vi "CH_LM Calibration Password.vi"(0 "Meter Index":i32, 2 "Password":string, 5 "error in (no error)":errorcluster, 7 "Timeout / ms (3000)":i32=3000, 9 "Lock Timeout / ms (1000)":i32=1000) -> (11 "Lock timed out":bool, 14 "Meter Index":i32, 19 "error out":errorcluster)   [LabVIEW 2012, in "CH_LM.lvlib"]
doc: "This command will enable calibration functionality by using a password. Calibration functionality will always be disabled after a power off/on cycle. Using the correct calibration password will enable calibration functionality. The password may be quoted or unquoted."
uses:
  CH_LM.lvlib
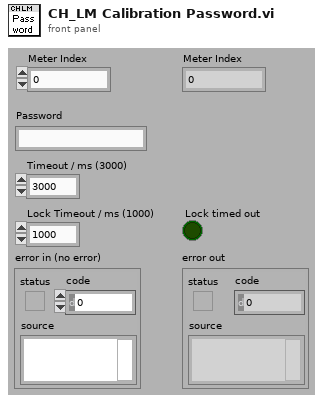
[diagram p1: front panel]
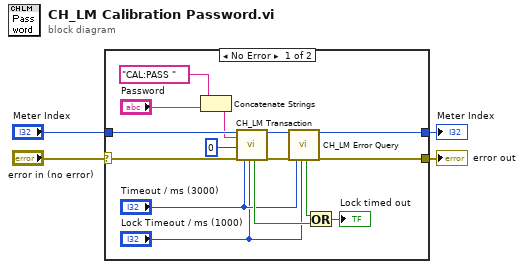
[diagram p0: block diagram]
diagram:
  n1 = case shown="No Error" "error in (no error)" {
    selector: "error in (no error)" -> [w19 w21]
    tunnel: [w14 w21] -> w4
    tunnel: "Meter Index" -> [w18 w20]
    tunnel: [w15 w20] -> w1
    frame No Error {
      n2 = Concatenate Strings("CAL:PASS ", "Password") -> (w5:string)
      n3 = call "CH_LM Transaction.vi"("Meter Index"=w18, "Command String"=w5, "NofStrings (-1:all)"=0, "error in (no error)"=w19, "Timeout / ms (3000)"="Timeout / ms (3000)", "Lock Timeout / ms (1000)"="Lock Timeout / ms (1000)") -> ("Lock timed out"=w12:bool, "Meter Index"=w17:i32, "error out"=w16:errorcluster)  [unwired: 11 out]
      n4 = call "CH_LM Error Query.vi"("Meter Index"=w17, "error in (no error)"=w16, "Timeout / ms (3000)"="Timeout / ms (3000)", "Lock Timeout / ms (1000)"="Lock Timeout / ms (1000)") -> ("Lock timed out"=w13:bool, "Meter Index"=w15:i32, "error out"=w14:errorcluster)  [unwired: 13 out]
      n5 = Or(x=w13, y=w12) -> (x .or. y?=→"Lock timed out":bool)
    }
    frame Error {
    }
  }
  "error out" <- w4
  "Meter Index" <- w1
